vi "FindEmptySubpanel.vi"(8 "error in (no error)":errorcluster, 10 "Match Index":i32, 11 "SMO.UI.MAUI in":refnum<class "MAUI.lvclass">) -> (0 "error out":errorcluster, 1 "Subpanel Index":i32, 2 "Ring Control":refnum<vi>, 3 "SMO.UI.MAUI out":refnum<class "MAUI.lvclass">, 4 "Empty Subpanel Exists?":bool)   [LabVIEW 2019, in "MAUI.lvclass"]
doc: "Compares the list of subpanels to the list of subpanels currently in use. Provides the index of the first empty subpanel it finds."
uses:
  MAUI.lvclass
  MAUI.lvclass/MAUI.ctl
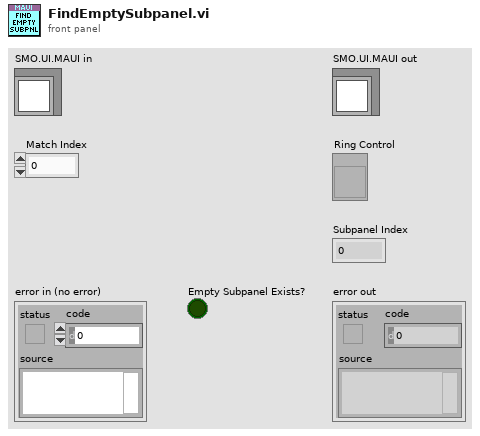
[diagram p1: front panel]
types:
  T1 = typedef "MAUI.lvclass/PanelData.ctl" = cluster{"SubPanel":refnum<vi>, "Ring":refnum<vi>, "Active":i32}
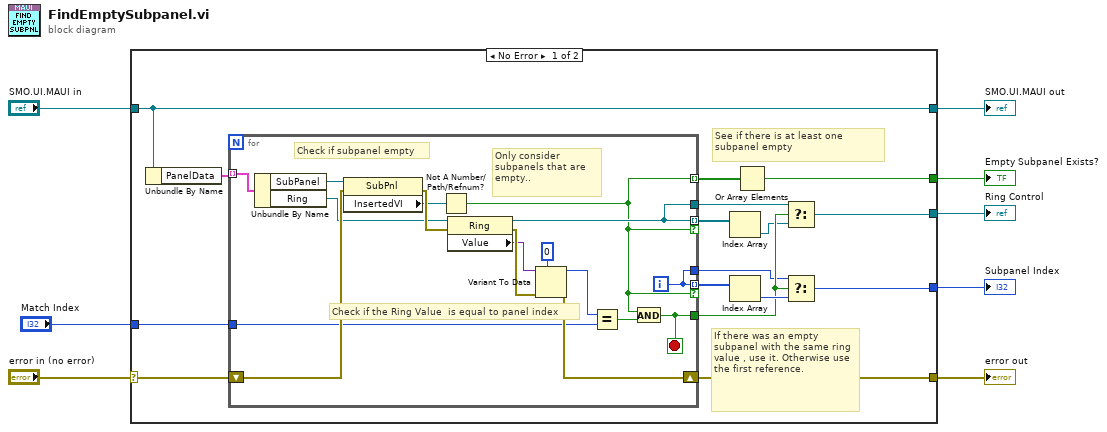
[diagram p0: block diagram]
diagram:
  n1 = case shown="No Error" "error in (no error)" {
    selector: "error in (no error)" -> [w24 w43]
    tunnel: [w23 w43] -> w7
    tunnel: [w22 w42] -> w5
    tunnel: "SMO.UI.MAUI in" -> [w22 w42]
    tunnel: "Match Index" -> [w20 _]
    tunnel: [w11 _] -> w3
    tunnel: [w10 _] -> w2
    tunnel: [w9 _] -> w1
    frame No Error {
      # "See if there is at least one subpanel empty"
      # "If there was an empty subpanel with the same ring value , use it. Otherwise use the first reference."
      n2 = Unbundle By Name(w22) -> ("PanelData"=w21:T1[])
      n3 = for {
        tunnel: w21 -> [w37] mode=indexing
        shift-right: [w39] -> w23
        shift-left: w24 -> [w38]
        tunnel: [w33] -> w16
        tunnel: [w29] -> w18 mode=indexing if=w27
        tunnel: w20 -> [w31]
        tunnel: [w30] -> w19 mode=indexing if=w27
        tunnel: [w30] -> w15
        tunnel: [w29] -> w13
        tunnel: [w27] -> w12 mode=indexing
        i -> [w29]
        stop <- w33 stop-if-true
        # "Only consider subpanels that are empty.."
        # "Check if the Ring Value  is equal to panel index"
        # "Check if subpanel empty"
        n4 = Unbundle By Name(w37) -> ("SubPanel"=w36:refnum<vi>, "Ring"=w26:refnum<vi>)
        n5 = property on="Property Node" class="SubPnl"(reference=w36, error in=w38) -> (error out=w41:errorcluster, "InsertedVI"=w25:refnum<vi>)  [unwired: 1 out]
        n6 = Not A Number/Path/Refnum?(number/path/refnum=w25) -> (NaN/Path/Refnum?=w27:bool)
        n7 = property on="Property Node" class="Ring"(reference=w26, error in=w41) -> (reference out=w30:refnum<vi>, error out=w40:errorcluster, "Value"=w28:variant)
        n8 = Variant To Data(error in=w40, type=0, Variant=w28) -> (data=w32:i32, error out=w39:errorcluster)
        n9 = Equal?(x=w32, y=w31) -> (x = y?=w34:bool)
        n10 = And(x=w27, y=w34) -> (x .and. y?=w33:bool)
      }
      n11 = Index Array(array=w19) -> (element=w14:refnum<vi>)  [unwired: 1 in]
      n12 = Index Array(array=w18) -> (element=w17:i32)  [unwired: 1 in]
      n13 = Or Array Elements(Boolean array=w12) -> (logical OR=w11:bool)
      n14 = Select(t=w15, s=w16, f=w14) -> (s? t:f=w9:refnum<vi>)
      n15 = Select(t=w13, s=w16, f=w17) -> (s? t:f=w10:i32)
    }
    frame Error {
    }
  }
  "error out" <- w7
  "SMO.UI.MAUI out" <- w5
  "Empty Subpanel Exists?" <- w3
  "Ring Control" <- w1
  "Subpanel Index" <- w2
